vi "SetStringGlobalVariables.vi"(8 "error in (no error)":errorcluster, 9 "values":string[](array[string]), 10 "varNumber":i32, 11 "controller in":refnum<k24>) -> (0 "error out":errorcluster, 3 "controller out":refnum<k24>)   [LabVIEW 2010]
uses:
  c:/aerotech/controller/dev/A3200/pc/labview/2010/bin/Aerotech.A3200.dll
  bin/Aerotech.A3200.dll
  c:/aerotech/controller/dev/A3200/pc/labview/2010/bin/Aerotech.A3200.LabVIEW.dll
  bin/Aerotech.A3200.LabVIEW.dll
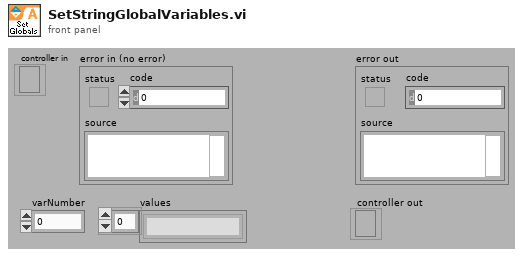
[diagram p1: front panel]
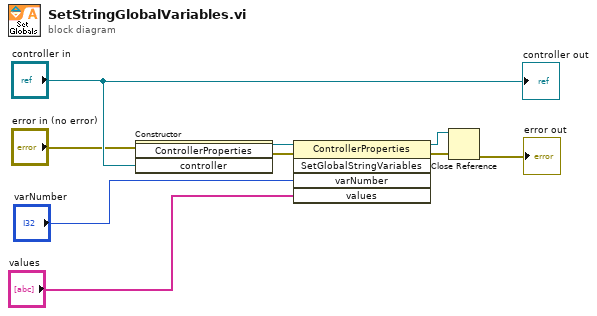
[diagram p0: block diagram]
diagram:
  n1 = constructor class="ControllerProperties"(error in="error in (no error)", "controller"="controller in") -> (reference out=w9:refnum<k24>, error out=w8:errorcluster)  [unwired: 2 in, 2 out]
  n2 = invoke class="ControllerProperties" method="SetGlobalStringVariables"(reference=w9, error in=w8, "varNumber"="varNumber", "values"="values") -> (reference out=w2:refnum<k24>, error out=w3:errorcluster)  [unwired: 1 in, 3 out]
  n3 = Close Reference(reference=w2, error in (no error)=w3) -> (error out=→"error out":errorcluster)
  "controller out" <- "controller in"
